vi "Print.vi"(8 "error in (no error)":errorcluster, 11 "Message Double in":refnum<class "Message Double.lvclass">) -> (0 "error out":errorcluster, 2 "String":string, 3 "Message Double out":refnum<class "Message Double.lvclass">)   [LabVIEW 2016, in "Stream Mediator.lvlib" / "Message Double.lvclass"]
doc: "--\nCopyright © 2017 Composed SystemsI All rights reserved.\n\nAuthor: Jon McBee <jon.mcbee@composed.io>\n\nThis library is provided \"AS IS\" ,WITHOUT WARRANTIES OR\nCONDITIONS OF ANY KIND, either express or implied.\n\nComposed Systems -- composed.io\n\nStream 0.0.1.1\nJon McBee - Composed Systems\nCopyright (c) 2017, Composed Systems"
uses:
  <userlib>/Composed Systems/Stream/Mediator/Classes/Message Double/Message Double.lvclass
  C:/Program Files (x86)/National Instruments/LabVIEW 2016/user.lib/Composed Systems/Stream/Mediator/Classes/Message Interface/Message Interface.lvclass
  <userlib>/Composed Systems/Stream/Mediator/Classes/Message Double/Message Double.lvclass/Message Double.ctl
  <vilib>/addons/_JKI.lib/Serialization/JSON/JKI JSON Serialization.lvlib
  <userlib>/Composed Systems/Stream/Mediator/Classes/Message Interface/Message Interface.lvclass
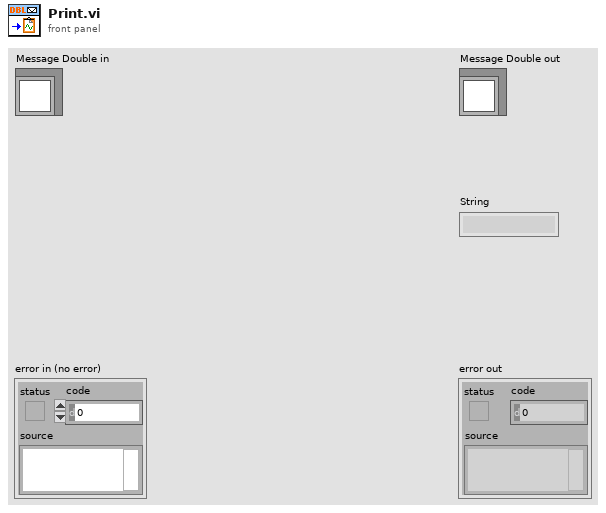
[diagram p1: front panel]
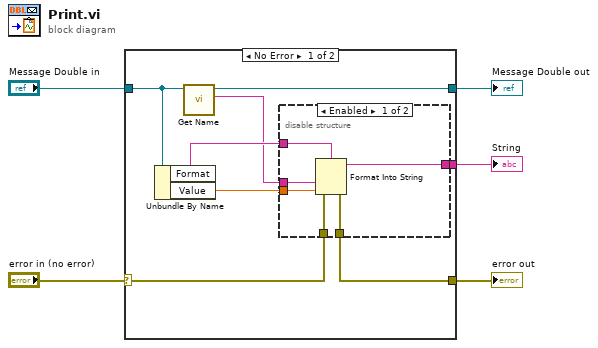
[diagram p0: block diagram]
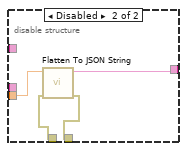
[diagram p2: hidden frame]
diagram:
  n1 = case shown="No Error" "error in (no error)" {
    selector: "error in (no error)" -> [w8 w24]
    tunnel: [w7 w24] -> w4
    tunnel: [w12 w25] -> w2
    tunnel: "Message Double in" -> [w13 w25]
    tunnel: [w6 _] -> w1
    frame No Error {
      n2 = Unbundle By Name(w13) -> ("Format"=w11:string, "Value"=w10:dbl)
      n3 = call <userlib>:"Get Name.vi"("Message Interface in"=w13) -> ("Name"=w9:string, "Message Interface out"=w12:refnum<class "Message Double.lvclass">)  [unwired: 8 in, 1 out]
      n4 = disable-structure shown="Enabled" {
        disable-tunnel: w11 -> [w19 _]
        disable-tunnel: w10 -> [w18 w21]
        disable-tunnel: w9 -> [w17 _]
        disable-tunnel: w8 -> [w16 w23]
        disable-tunnel: [w15 w22] -> w7
        disable-tunnel: [w14 w20] -> w6
        frame Enabled {
          n5 = Format Into String(format string=w19, error in=w16, w17, w18) -> (resulting string=w14:string, error out=w15:errorcluster)  [unwired: 1 in]
        }
        frame Disabled {
          n6 = call <vilib>:"Flatten To JSON String.vi"("error in (no error)"=w23, "Variant"=w21) -> ("error out"=w22:errorcluster, "JSON String"=w20:string)  [unwired: 8 in]
        }
      }
    }
    frame Error {
    }
  }
  "error out" <- w4
  "Message Double out" <- w2
  "String" <- w1
